vi "SMS Image Preview.vi"(7 "Calling VI Ref":refnum<vi>) -> ()   [LabVIEW 2016]
uses:
  <vilib>/Utility/miscctls.llb/LVPointTypeDef.ctl
  Hardware Configuration/Hardware Configuration Controls/Device Function.ctl
  SMS Image Preview Type Defs/SMS Image Preview Notifier Type.ctl
  SMS Image Preview Type Defs/SMS Image Preview Actions.ctl
  <vilib>/vision/Image Controls.llb/IMAQ Image.ctl
  Device Library/Cameras/Hamamatsu/Orca Flash/Orca Flash Controls/Orca Flash Actions.ctl
  Hardware Configuration/Hardware Configuration Controls/Device Type.ctl
  Device Library/FPGA/FPGA Controls/FPGA Action.ctl
  Device Library/Cameras/Camera Controls/Camera IMAQ Key Info.ctl
  Device Library/Lasers/Laser Controls/Laser Actions.ctl
  Device Library/Lasers/Laser Controls/Laser Settings.ctl
  Device Library/Lasers/Laser Controls/Laser Parameters.ctl
  <vilib>/Analysis/baseanly.llb/Mean (DBL).vi
  <vilib>/vision/NI_Vision_Development_Module.lvlib
  <vilib>/Analysis/NI_AALBase.lvlib
panel:
  in  "YOffset":i32
  in  "XOffset":i32
  in  "Angle (degrees)":sgl format="%.2f"
  out "Current Emitter No.":u16
  in  "Duration":u32 max=65535 step=1
  in  "P Const.":dbl=0.5
  in  "Target Emitter No.":u16=3
  in  "Lock Density":bool
  in  "Average Frame No.":i32=100
  in  "Edge Size":i32=12
  in  "Use Quadrant":bool
  in  "Reset Plot":bool
  out "Blink No. vs. Time":cluster{dbl[], u16[]}(graph)
  in  "Accumulate":bool
  in  "Blink Sensitivity":sgl=10.0
  in  "Image Display":bool
  in  "SMS Preview":bool
  in  "Camera ROI":bool
  in  "Camera":i32(ring) items=["Hamamatsu-Camera-Primary-0"]
  in  "Quit":bool
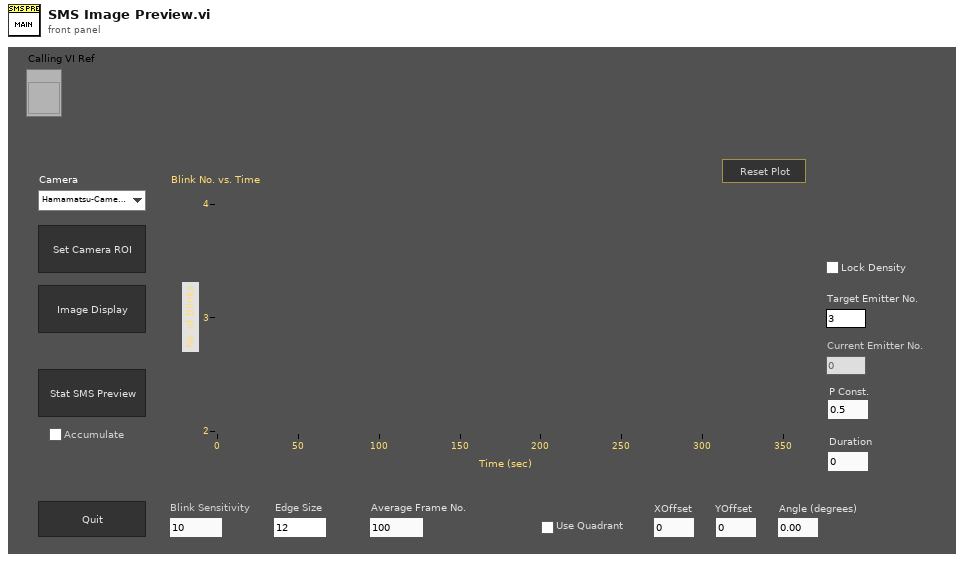
[diagram p1: front panel]
types:
  T1 = typedef "Image Type" = u32
  T2 = typedef "FPGA Action.ctl" = enum16{"Set Laser Mode", "Set Sequence", "Set Duration", "Write Check", "Idle", "Quit"}
  T3 = typedef "Device Function.ctl" = enum16{"Primary", "Secondary", "Overview", "Wide Field Drift Correction", "642 nm Excitation", "560 nm Excitation", "940 nm Excitation", "546 nm Excitation", "488 nm Excitation", "405 nm Excitation", "Objective Drift Correction", "4Pi Focus Lock", "4Pi Objective Lock", "Objective XY", "Objective Z", "Sample XY", "Sample Coarse Z", "Sample Z", "4Pi Lower", "4Pi Upper", "Em Small", "Em Large", "Ex Small", "Ex Large", "Mojo", "Adj Cavity", "Line Scanning", "Alert"}
  T4 = typedef "Device Type.ctl" = enum16{"AOTF", "Camera", "Deformable Mirror", "Laser", "Flip Mirror", "Shutter", "Stage", "Waveform", "FPGA", "Email"}
  T5 = enum8{"Enabled", "Disabled", "Disabled and Grayed Out"}
  T6 = typedef "Orca Flash Actions.ctl" = enum16{"IDLE", "PREVIEW", "RECORD", "Send Trigger", "SOFT TRIGGER", "Record Settings", "SETPARAM", "GETPARAM", "SETROI", "GETROI", "PROGRESSIVE MODE", "AREA MODE", "STATUS", "QUIT"}
  T7 = typedef "SMS Image Preview Actions.ctl" = enum16{"Idle", "Start SMS Preview", "Get Image", "Get Quad", "Sum Quad", "Convolve and Threshold", "Subtract > Dilate", "And Image", "Remove Edge", "Update Plot", "Update Duration", "Abort", "Exit Loop", "Quit"}
  T8 = typedef "SMS Image Preview Notifier Type.ctl" = cluster{"Action":T7, "Camera Notifier Name":string, "Camera Image (U16)":T9, "Camera ROI":cluster{"Global Rectangle":i32[], "Contours":cluster{"Contour Type":u32, "ROI Type":u32, "Points":i32[]}[]}, "SMS Preview (U16)":T9, "Camera ROI (U16)":T9, "Threshold (U16)":T9, "Subtracted > Dilated (U16)":T9, "And Image (U16)":T9, "Camera ROI (SGL)":T9, "Conv 5 x 5 (SGL)":T9, "Conv 11 x 11 (SGL)":T9, "Subtracted (SGL)":T9, "Dilated (SGL)":T9, "Subtracted > Dilated (SGL)":T9, "Ones 5 x 5":sgl[][], "Ones 11 x 11":sgl[][], "Ones 7 x 7":i32[][], "Quads":T9[], "Edge Removed (U16)":T9, "Laser Notifier Name":string, "FPGA Notifier Name":string, "Duration":u32, "Quad 3 TM":T9}
  T9 = typedef "IMAQ Image.ctl" = refnum<image>
  T10 = enum16{"Always On", "Always Off", "Off While Running"}
  T11 = typedef "LVPointTypeDef.ctl" = cluster{"Horizontal":i16, "Vertical":i16}
  T12 = typedef "Camera IMAQ Key Info.ctl" = cluster{"Frame":u32, "Sensor Height":i32, "Sensor Width":i32, "ROI Height":i32, "ROI Width":i32, "ROI Enable?":bool, "Bit per Pixel":u8}
  T13 = enum32{"Average", "Min", "Max", "Clear  if < ", "Clear  if < or =", "Clear  if =", "Clear  if > or =", "Clear  if >"}
  T14 = enum32{"AutoM", "Close", "Dilate", "Erode", "Gradient", "Gradient in", "Gradient out", "HitMiss", "Open", "PClose", "POpen", "Thick", "Thin"}
  T15 = enum32{"Invalid", "Standard", "Closed", "Hidden", "Minimized", "Maximized"}
  T16 = cluster{"Global Rectangle":i32[], "Contours":cluster{"Contour Type":u32, "ROI Type":u32, "Points":i32[]}[]}
  T17 = typedef "Laser Parameters.ctl" = enum16{"Wavelength (nm)", "Pulsing?", "Rep. Rate", "External Control", "Enable Fine", "Fine A", "Fine B", "Channel No."}
  T18 = typedef "Laser Settings.ctl" = cluster{"Laser Parameters":T17, "Value":dbl}
  T19 = typedef "Laser Actions.ctl" = enum16{"Error Check", "Set On/Off", "Set Power", "Set Parameter", "Get Power", "Get Status", "Get Parameter", "Quit"}
  T20 = cluster{"histogram":u32[], "Minimal Value":sgl, "Maximal Value":sgl, "Starting Value":sgl, "Interval Width":sgl, "Mean Value":sgl, "Standard  Variation":sgl, "Area (pixels)":i32}
  T21 = typedef "LVRectTypeDef.ctl" = cluster{"Left":i16, "Top":i16, "Right":i16, "Bottom":i16}
  T22 = typedef "LVBoundsTypeDef.ctl" = cluster{"Width":u32, "Height":u32}
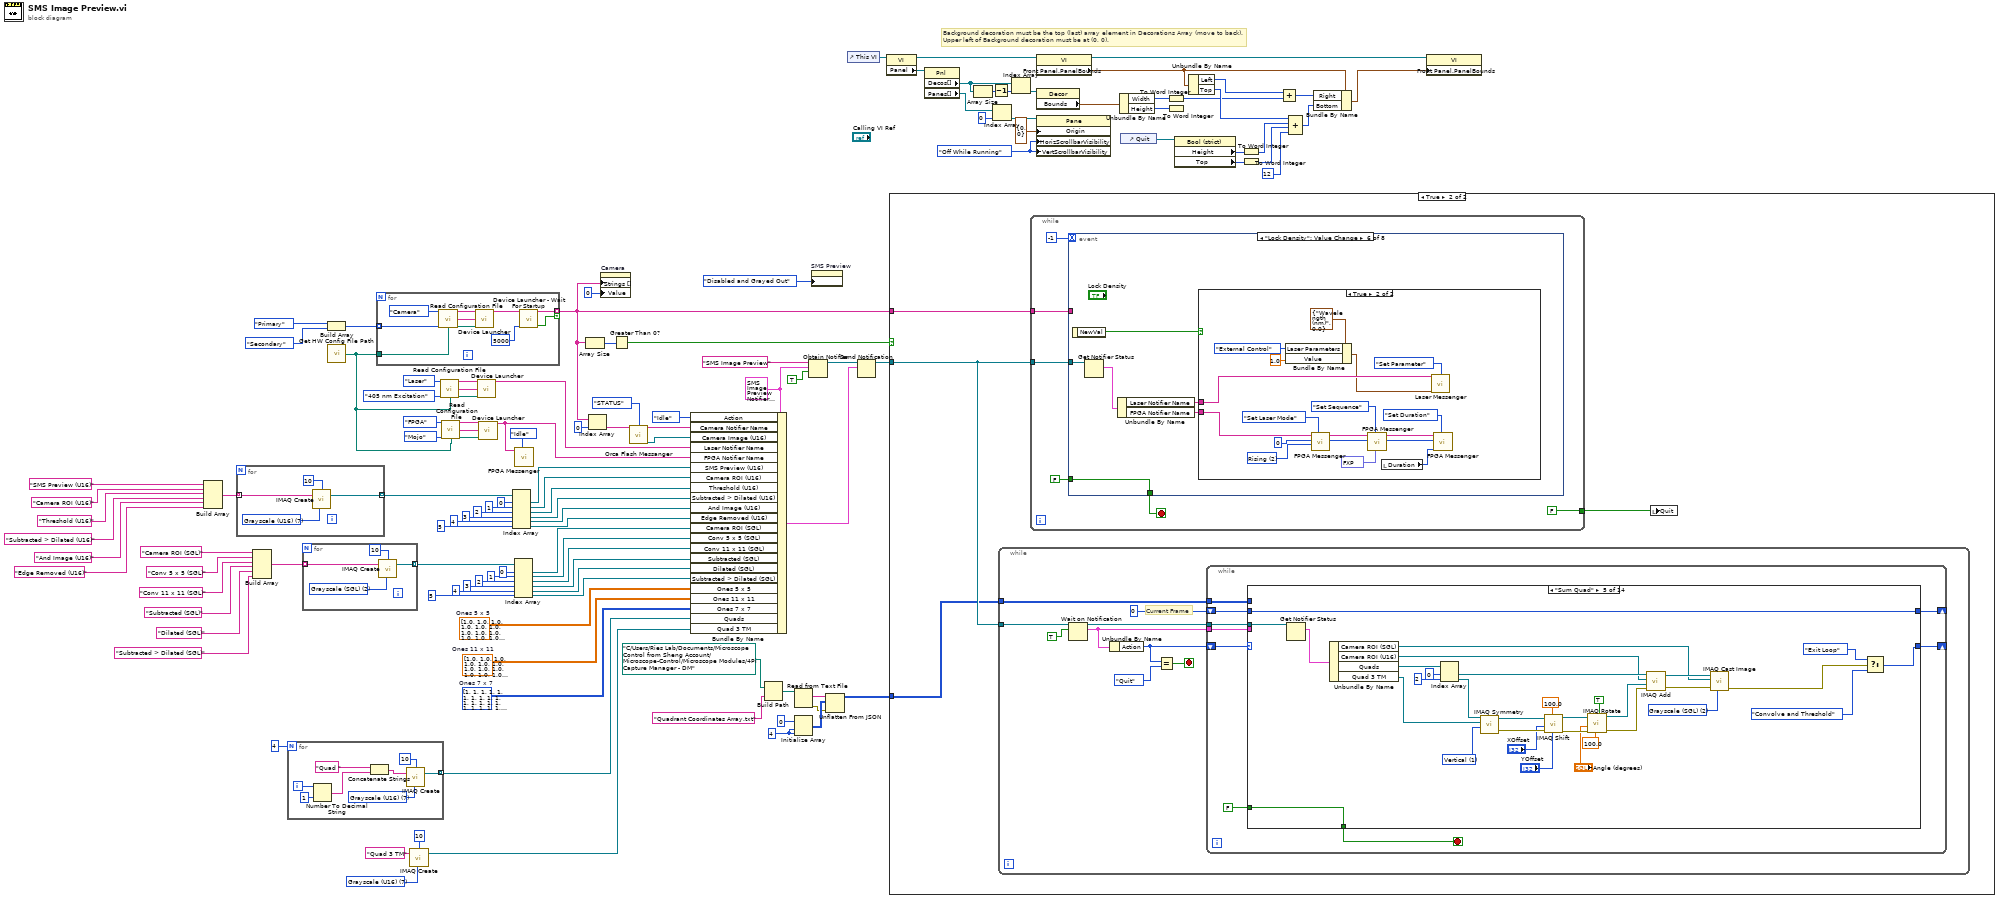
[diagram p0: block diagram]
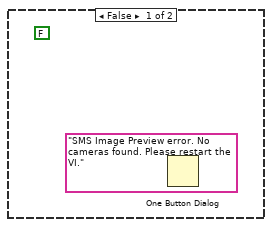
[diagram p2: hidden frame]
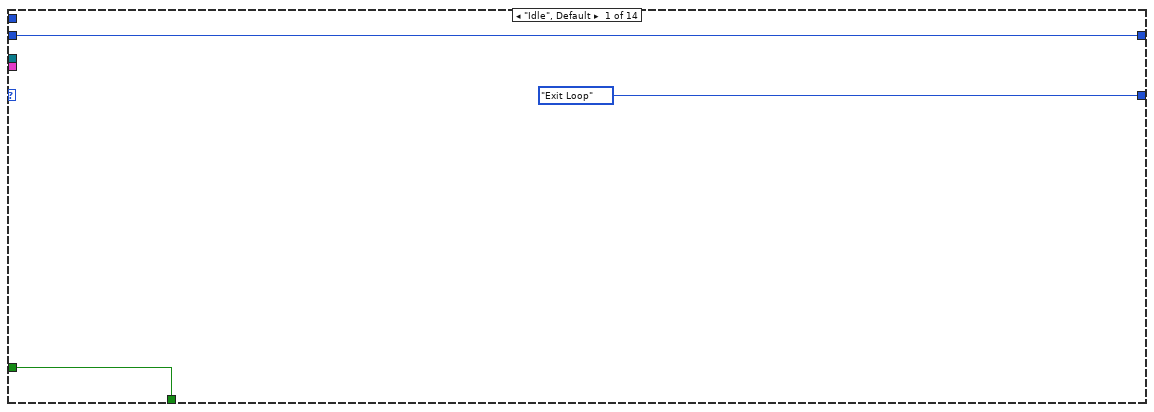
[diagram p3: hidden frame]
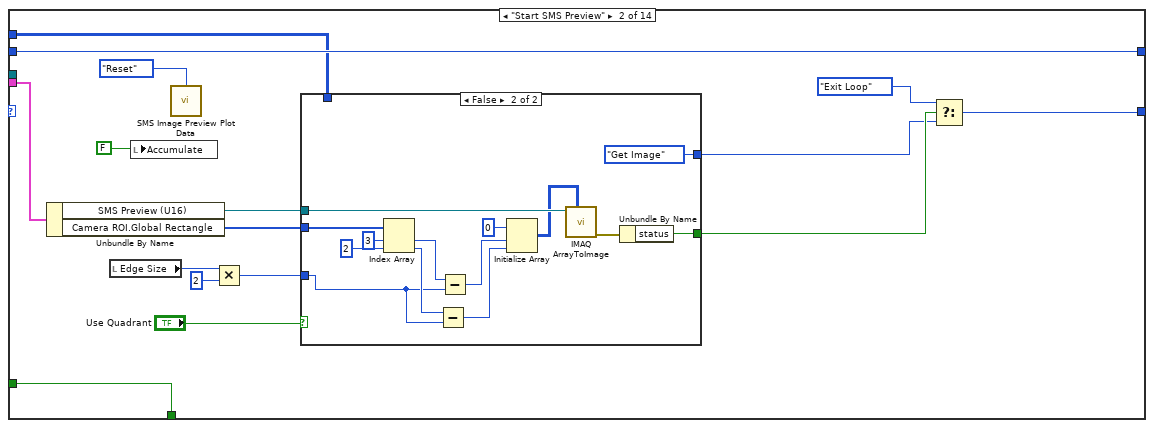
[diagram p4: hidden frame]
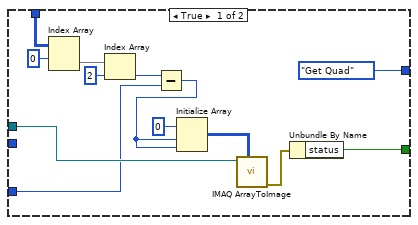
[diagram p5: hidden frame]
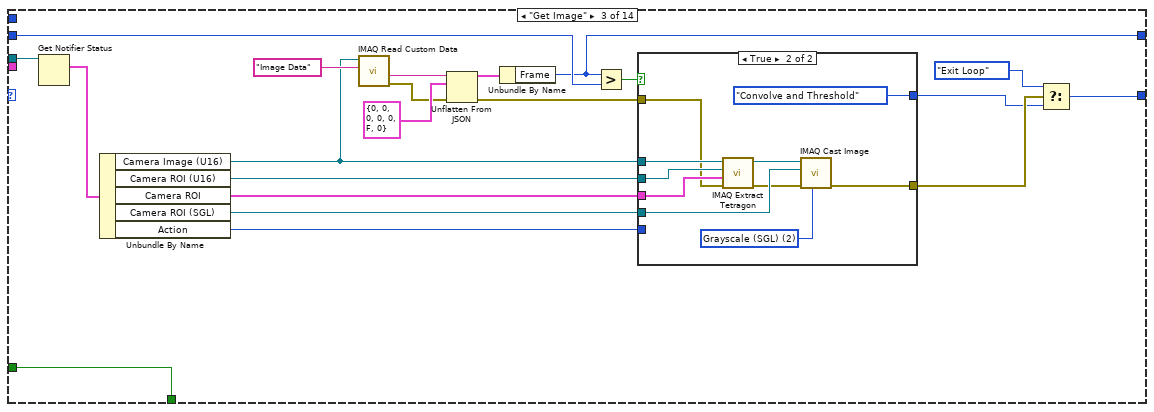
[diagram p6: hidden frame]
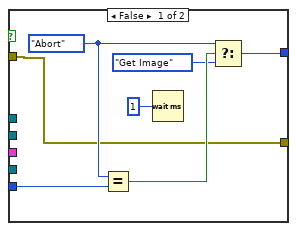
[diagram p7: hidden frame]
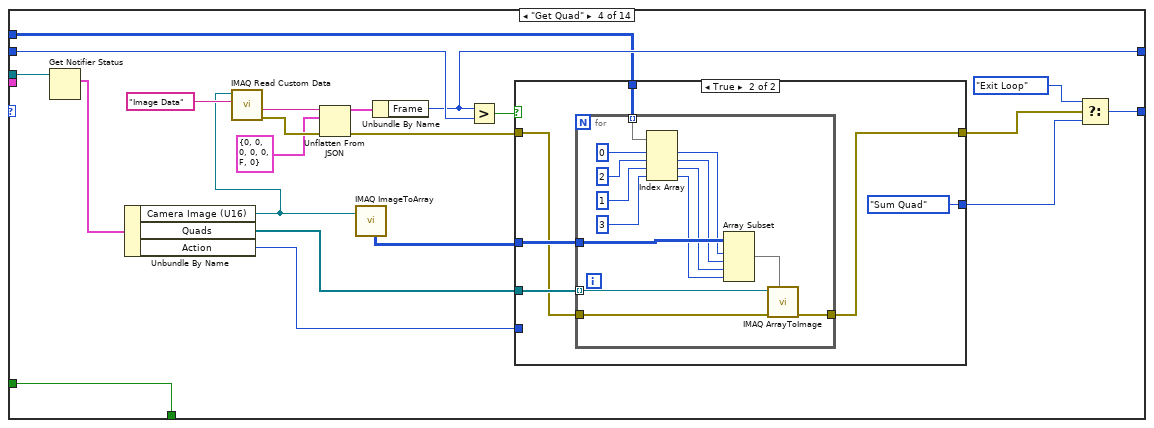
[diagram p8: hidden frame]
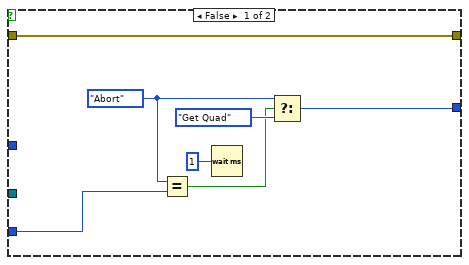
[diagram p9: hidden frame]
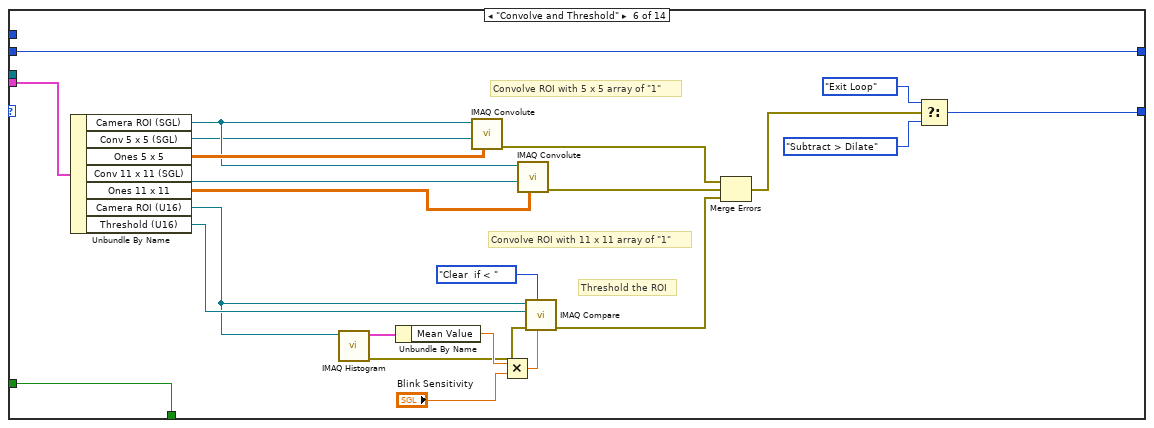
[diagram p10: hidden frame]
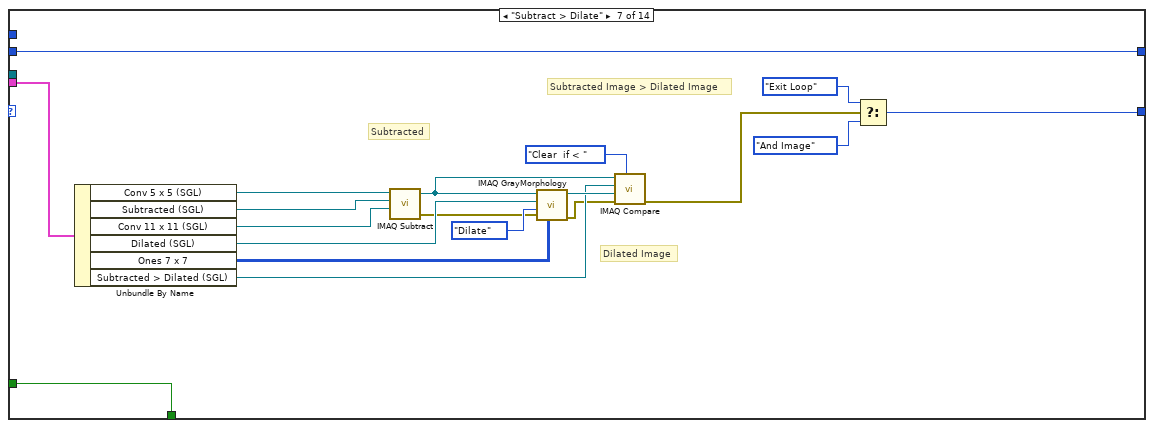
[diagram p11: hidden frame]
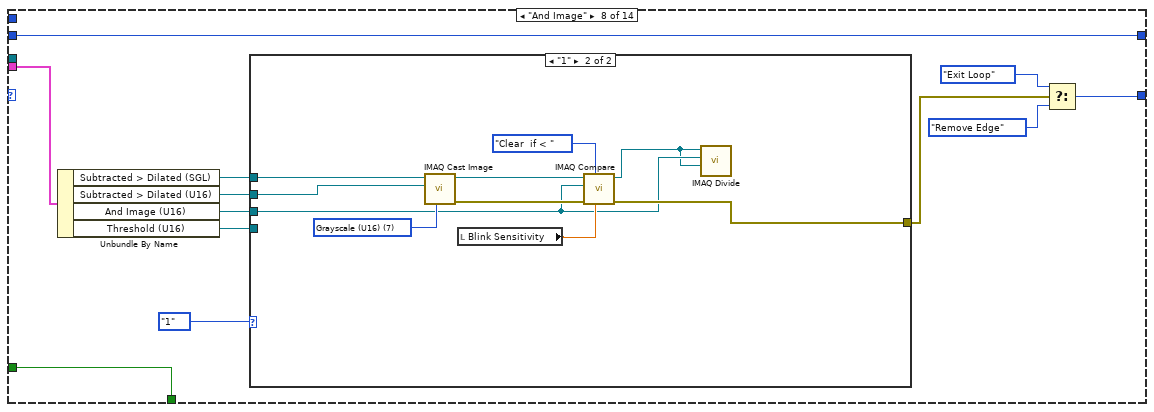
[diagram p12: hidden frame]
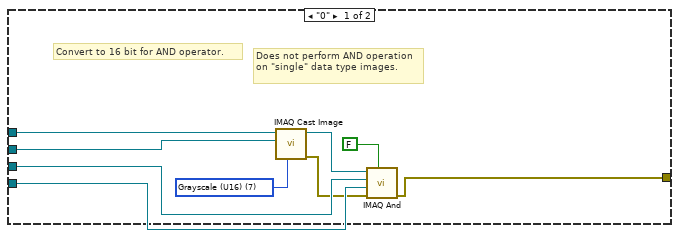
[diagram p13: hidden frame]
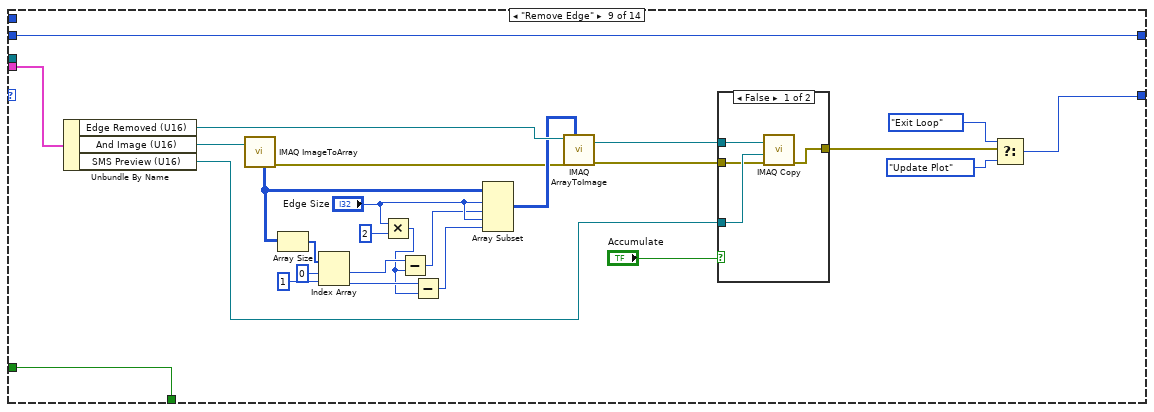
[diagram p14: hidden frame]
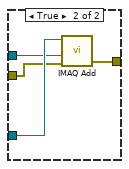
[diagram p15: hidden frame]
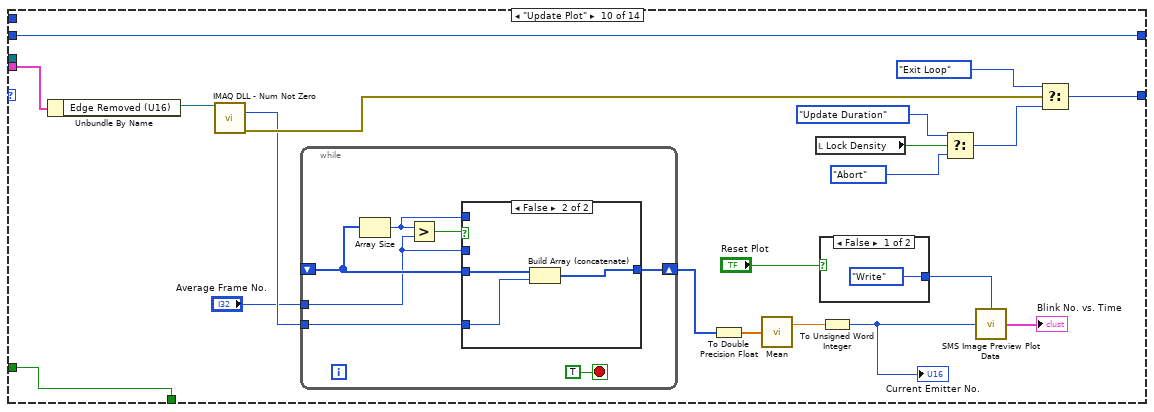
[diagram p16: hidden frame]
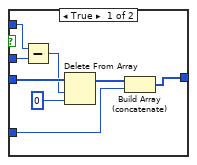
[diagram p17: hidden frame]
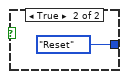
[diagram p18: hidden frame]
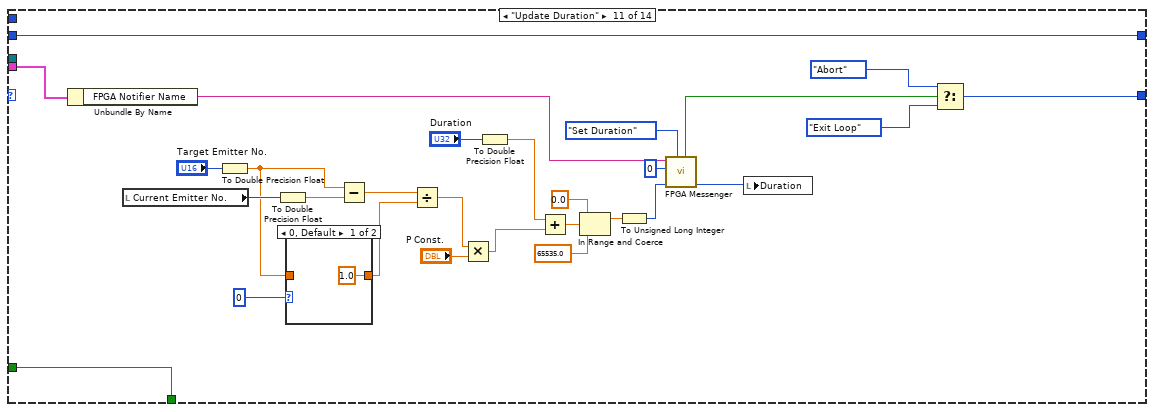
[diagram p19: hidden frame]
diagram:
  w5 = T1 7 items=["Grayscale (U8)", "Grayscale (I16)", "Grayscale (SGL)", "Complex (CSG)", "RGB (U32)", "HSL (U32)", "RGB (U64)", "Grayscale (U16)"] ("Image Type")
  w26 = 4 ("dimension size")
  w37 = i32[][] [[1, 1, 1, 1, 1, 1, 1], [1, 1, 1, 1, 1, 1, 1], [1, 1, 1, 1, 1, 1, 1], [1, 1, 1, 1, 1, 1, 1], [1, 1, 1, 1, 1, 1, 1], [1, 1, 1, 1, 1, 1, 1], [1, 1, 1, 1, 1, 1, 1]]  # Ones 7 x 7
  w38 = sgl[][] [[1.0, 1.0, 1.0, 1.0, 1.0, 1.0, 1.0, 1.0, 1.0, 1.0, 1.0], [1.0, 1.0, 1.0, 1.0, 1.0, 1.0, 1.0, 1.0, 1.0, 1.0, 1.0], [1.0, 1.0, 1.0, 1.0, 1.0, 1.0, 1.0, 1.0, 1.0, 1.0, 1.0], [1.0, 1.0, 1.0, 1.0, 1.0, 1.0, 1.0, 1.0, 1.0, 1.0, 1.0], [1.0, 1.0, 1.0, 1.0, 1.0, 1.0, 1.0, 1.0, 1.0, 1.0, 1.0], [1.0, 1.0, 1.0, 1.0, 1.0, 1.0, 1.0, 1.0, 1.0, 1.0, 1.0], [1.0, 1.0, 1.0, 1.0, 1.0, 1.0, 1.0, 1.0, 1.0, 1.0, 1.0], [1.0, 1.0, 1.0, 1.0, 1.0, 1.0, 1.0, 1.0, 1.0, 1.0, 1.0], [1.0, 1.0, 1.0, 1.0, 1.0, 1.0, 1.0, 1.0, 1.0, 1.0, 1.0], [1.0, 1.0, 1.0, 1.0, 1.0, 1.0, 1.0, 1.0, 1.0, 1.0, 1.0], [1.0, 1.0, 1.0, 1.0, 1.0, 1.0, 1.0, 1.0, 1.0, 1.0, 1.0]]  # Ones 11 x 11
  w39 = sgl[][] [[1.0, 1.0, 1.0, 1.0, 1.0], [1.0, 1.0, 1.0, 1.0, 1.0], [1.0, 1.0, 1.0, 1.0, 1.0], [1.0, 1.0, 1.0, 1.0, 1.0], [1.0, 1.0, 1.0, 1.0, 1.0]]  # Ones 5 x 5
  w34 = T8 {"Action"=enum."Idle", "Camera Notifier Name"="", "Camera Image (U16)"=refnum, "Camera ROI"={"Global Rectangle"=[], "Contours"=[]}, "SMS Preview (U16)"=refnum, "Camera ROI (U16)"=refnum, "Threshold (U16)"=refnum, "Subtracted > Dilated (U16)"=refnum, "And Image (U16)"=refnum, "Camera ROI (SGL)"=refnum, "Conv 5 x 5 (SGL)"=refnum, "Conv 11 x 11 (SGL)"=refnum, "Subtracted (SGL)"=refnum, "Dilated (SGL)"=refnum, "Subtracted > Dilated (SGL)"=refnum, "Ones 5 x 5"=[], "Ones 11 x 11"=[], "Ones 7 x 7"=[], "Quads"=[], "Edge Removed (U16)"=refnum, "Laser Notifier Name"="", "FPGA Notifier Name"="", "Duration"=0, "Quad 3 TM"=refnum} ("SMS Image Preview Notifier Type")
  w104 = T10."Off While Running" ("Vertical Scrollbar Visibility")
  # "Background decoration must be the top (last) array element in Decorations Array (move to back).\nUpper left of Background decoration must be at (0, 0)."
  n1 = Build Array("SMS Preview (U16)" ("Image Name"), "Camera ROI (U16)" ("Image Name"), "Threshold (U16)" ("Image Name"), "Subtracted > Dilated (U16)" ("Image Name"), "And Image (U16)" ("Image Name"), "Edge Removed (U16)" ("element")) -> (w49:string[])
  n2 = for {
    tunnel: w49 -> [w123] mode=indexing
    tunnel: [w122] -> w50 mode=indexing
    w124 = T1 7 items=["Grayscale (U8)", "Grayscale (I16)", "Grayscale (SGL)", "Complex (CSG)", "RGB (U32)", "HSL (U32)", "RGB (U64)", "Grayscale (U16)"] ("Image Type")
    n3 = call "IMAQ Create"("Border Size"=10, "Image Name"=w123, "Image Type"=w124) -> ("New Image"=w122:T9)  [unwired: 2 in, 1 out]
  }
  n4 = Build Array("Camera ROI (SGL)" ("Image Name"), "Conv 5 x 5 (SGL)" ("Image Name"), "Conv 11 x 11 (SGL)" ("Image Name"), "Subtracted (SGL)" ("Image Name"), "Dilated (SGL)" ("Image Name"), "Subtracted > Dilated (SGL)" ("Image Name")) -> (w69:string[])
  n5 = for {
    N: 4 -> [_]
    tunnel: [w131] -> w33 mode=indexing
    i -> [w130]
    w133 = T1 7 items=["Grayscale (U8)", "Grayscale (I16)", "Grayscale (SGL)", "Complex (CSG)", "RGB (U32)", "HSL (U32)", "RGB (U64)", "Grayscale (U16)"] ("Image Type")
    n6 = Number To Decimal String(number=w130, width (-)=i16 1) -> (decimal integer string=w127:string)
    n7 = Concatenate Strings("Quad " ("Image Name"), w127) -> (w126:string)
    n8 = call "IMAQ Create"("Border Size"=10, "Image Name"=w126, "Image Type"=w133) -> ("New Image"=w131:T9)  [unwired: 2 in, 1 out]
  }
  n9 = for {
    tunnel: w69 -> [w135] mode=indexing
    tunnel: [w134] -> w68 mode=indexing
    w136 = T1 2 items=["Grayscale (U8)", "Grayscale (I16)", "Grayscale (SGL)", "Complex (CSG)", "RGB (U32)", "HSL (U32)", "RGB (U64)", "Grayscale (U16)"] ("Image Type")
    n10 = call "IMAQ Create"("Border Size"=10, "Image Name"=w135, "Image Type"=w136) -> ("New Image"=w134:T9)  [unwired: 2 in, 1 out]
  }
  n11 = Build Array(Device_Function."Primary" ("Device Function"), Device_Function."Secondary" ("Device Function")) -> (w90:T3[])
  n12 = call "Get HW Config File Path.vi"() -> ("File Path"=w8:path)  [unwired: 14 in, 1 out]
  n13 = for {
    tunnel: w90 -> [w143] mode=indexing
    tunnel: w8 -> [w142]
    tunnel: [w140] -> w80 mode=indexing if=w139
    n14 = call "Read Configuration File.vi"("Device Type"=Device_Type."Camera", "Device Function"=w143, "Config File Path"=w142) -> ("Unique Notifier Name"=w145:string, "Device Ports/IDs/Channels"=w147:string[], "Device Engine Path"=w146:path)  [unwired: 9 in, 1 out]
    n15 = call "Device Launcher.vi"("Notifier Name"=w145, "Device Ports/IDs/Channels"=w147, "Device Engine Path"=w146) -> ("Notifier Name"=w141:string)  [unwired: 11 in, 1 out]
    n16 = call "Device Launcher - Wait For Startup.vi"("Notifier Name"=w141, "Wait Time (ms)"=5000) -> ("Notifier Name (Dup)"=w140:string, "Running?"=w139:bool)  [unwired: 12 in]
  }
  n17 = call "IMAQ Create"("Border Size"=10, "Image Name"="Quad 3 TM", "Image Type"=w5) -> ("New Image"=w2:T9)  [unwired: 2 in, 1 out]
  n18 = call "Read Configuration File.vi"("Device Type"=Device_Type."Laser", "Device Function"=Device_Function."405 nm Excitation", "Config File Path"=w8) -> ("Unique Notifier Name"=w17:string, "Device Ports/IDs/Channels"=w16:string[], "Device Engine Path"=w15:path)  [unwired: 9 in, 1 out]
  n19 = call "Read Configuration File.vi"("Device Type"=Device_Type."FPGA", "Device Function"=Device_Function."Mojo", "Config File Path"=w8) -> ("Unique Notifier Name"=w11:string, "Device Ports/IDs/Channels"=w10:string[], "Device Engine Path"=w9:path)  [unwired: 9 in, 1 out]
  n20 = call "Device Launcher.vi"("Notifier Name"=w17, "Device Ports/IDs/Channels"=w16, "Device Engine Path"=w15) -> ("Notifier Name"=w14:string)  [unwired: 11 in, 1 out]
  n21 = call "Device Launcher.vi"("Notifier Name"=w11, "Device Ports/IDs/Channels"=w10, "Device Engine Path"=w9) -> ("Notifier Name"=w7:string)  [unwired: 11 in, 1 out]
  n22 = Index Array(array=w50, index #1=0 ("index"), index #2=1 ("index"), index #3=2 ("index"), index #4=3 ("index"), index #5=4 ("index"), index #6=5 ("index")) -> (element #1=w48:T9, element #2=w47:T9, element #3=w46:T9, element #4=w22:T9, element #5=w21:T9, element #6=w20:T9)
  n23 = Index Array(array=w68, index #1=0 ("index"), index #2=1 ("index"), index #3=2 ("index"), index #4=3 ("index"), index #5=4 ("index"), index #6=5 ("index")) -> (element #1=w45:T9, element #2=w44:T9, element #3=w43:T9, element #4=w42:T9, element #5=w41:T9, element #6=w40:T9)
  n24 = call "FPGA Messenger.vi"("FPGA Action"=FPGA_Action."Idle", "Notifier Name"=w7) -> ()  [unwired: 4 in, 6 out]
  n25 = Array Size(array=w80) -> (size(s)=w89:i32)
  n26 = Index Array(array=w80, index=0) -> (element=w78:string)
  n27 = property on="Camera" class="Ring (strict)"("Strings []"=w80, "Value"=0) -> ()  [unwired: 2 in, 2 out]
  n28 = Greater Than 0?(x=w89) -> (x > 0?=w88:bool)
  n29 = call "Orca Flash Messanger.vi"("Notifier Name"=w78, "Camera Actions"=Orca_Flash_Actions."STATUS") -> ("Notifier Name Dup"=w77:string, "Image Ref"=w75:T9)  [unwired: 9 in, 3 out]
  n30 = Bundle By Name(cluster=w34, "Action"=SMS_Image_Preview_Actions."Idle", "Camera Notifier Name"=w77, "Camera Image (U16)"=w75, "Laser Notifier Name"=w14, "FPGA Notifier Name"=w7, "SMS Preview (U16)"=w48, "Camera ROI (U16)"=w47, "Threshold (U16)"=w46, "Subtracted > Dilated (U16)"=w22, "And Image (U16)"=w21, "Edge Removed (U16)"=w20, "Camera ROI (SGL)"=w45, "Conv 5 x 5 (SGL)"=w44, "Conv 11 x 11 (SGL)"=w43, "Subtracted (SGL)"=w42, "Dilated (SGL)"=w41, "Subtracted > Dilated (SGL)"=w40, "Ones 5 x 5"=w39, "Ones 11 x 11"=w38, "Ones 7 x 7"=w37, "Quads"=w33, "Quad 3 TM"=w2) -> (w81:T8)
  n31 = Build Path(base path=path "C:/Users/Ries Lab/Documents/Microscope Control from Sheng Account/Microscope-Control/Microscope Modules/4Pi Capture Manager - DM" ("path"), name or relative path="Quadrant Coordinates Array.txt") -> (appended path=w29:path)
  n32 = Read from Text File(file (use dialog)=w29) -> (text=w28:string, error out=w27:errorcluster)  [unwired: 3 in, 2 out]
  n33 = Initialize Array(0 ("element"), w26, w26) -> (w30:i32[][])
  n34 = Obtain Notifier(name (unnamed)="SMS Image Preview", notification data type=w34, create if not found? (T)=TRUE) -> (notifier out=w84:refnum<notifier>)  [unwired: 1 in, 2 out]
  n35 = property on="SMS Preview" class="Bool (strict)"("DisabledEnum"=T5."Disabled and Grayed Out" ("Disabled")) -> ()  [unwired: 2 in, 2 out]
  n36 = Unflatten From JSON(JSON string=w28, type and defaults=w30, error in (no error)=w27) -> (value=w25:i32[][])  [unwired: 4 in, 1 out]
  n37 = control-ref of="This VI"() -> (w96:refnum<vi>)
  n38 = Send Notification(notification=w81, notifier=w84) -> (notifier out=w82:refnum<notifier>)  [unwired: 1 in, 1 out]
  n39 = property class="VI"(reference=w96) -> (reference out=w105:refnum<vi>, "Panel"=w97:refnum<vi>)  [unwired: 1 in, 1 out]
  n40 = case shown="True" w88 {
    tunnel: w80 -> [_ w152]
    tunnel: w82 -> [_ w150]
    tunnel: w25 -> [_ w149]
    frame False {
      (unwired) FALSE
      n41 = One Button Dialog(message="SMS Image Preview error. No cameras found. Please restart the VI.") -> ()  [unwired: 1 in, 1 out]
    }
    frame True {
      n42 = while {
        tunnel: w150 -> [w161]
        tunnel: w149 -> [w153]
        stop <- w158 stop-if-true
        # "Current Frame"
        n43 = Wait on Notification(notifier=w161, ignore previous (F)=TRUE) -> (notifier out=w154:refnum<notifier>, notification=w156:T8)  [unwired: 2 in, 2 out]
        n44 = Unbundle By Name(w156) -> ("Action"=w157:T7)
        n45 = Equal?(x=w157, y=SMS_Image_Preview_Actions."Quit") -> (x = y?=w158:bool)
        n46 = while {
          shift-right: [w162] -> _
          shift-left: w157 -> [w170]
          tunnel: w156 -> [w169]
          shift-right: [w167] -> _
          shift-left: u32 0 -> [w168]
          tunnel: w154 -> [w166]
          tunnel: w153 -> [w163]
          stop <- w164 stop-if-true
          n47 = case shown="\"Sum Quad\"" w170 {
            tunnel: w169 -> [_ w187 _ _ _ w356 w375 w387 w423 w458 w498 _ _ _]
            tunnel: [SMS_Image_Preview_Actions."Exit Loop" ("y") w184 w219 w257 w312 w337 w358 w378 w415 w460 w500 w517 SMS_Image_Preview_Actions."Exit Loop" ("f") SMS_Image_Preview_Actions."Quit" ("f")] -> w162
            tunnel: w168 -> [w172 w189 w233 w266 w323 w357 w376 w388 w418 w461 w504 w522 w528 w545]
            tunnel: [w172 w189 w232 w265 w323 w357 w376 w388 w418 w461 w504 w522 w528 w545] -> w167
            tunnel: w166 -> [_ _ w227 w274 w324 _ _ _ _ _ _ w521 _ w542]
            tunnel: FALSE -> [w171 w188 w228 w275 w311 w347 w364 w382 w414 w453 w499 w515 _ _]
            tunnel: [w171 w188 w228 w275 w311 w347 w364 w382 w414 w453 w499 w515 TRUE TRUE] -> w164
            tunnel: w163 -> [_ w178 _ w256 _ _ _ _ _ _ _ _ _ _]
            frame "Idle", Default {
            }
            frame "Start SMS Preview" {
              n48 = Unbundle By Name(w187) -> ("SMS Preview (U16)"=w185:T9, "Camera ROI.Global Rectangle"=w186:i32[])
              n49 = local read "Edge Size"() -> (w176:i32)
              n50 = local write "Accumulate"(FALSE ("Accumulate")) -> ()
              n51 = call "SMS Image Preview Plot Data.vi"("Plot Data Actions"=enum16{"Read", "Write", "Reset"}."Reset") -> ()  [unwired: 14 in, 1 out]
              n52 = Multiply(x=w176, y=2) -> (x*y=w174:i32)
              n53 = case shown="False" "Use Quadrant" {
                tunnel: w186 -> [_ w216]
                tunnel: w185 -> [w193 w212]
                tunnel: [w199 w209] -> w183
                tunnel: [SMS_Image_Preview_Actions."Get Quad" ("y") SMS_Image_Preview_Actions."Get Image" ("y")] -> w179
                tunnel: w178 -> [w197 _]
                tunnel: w174 -> [w191 w204]
                frame True {
                  n54 = Index Array(array=w197, index (row)=0) -> (element=w195:i32[])  [unwired: 1 in]
                  n55 = Index Array(array=w195, index=2) -> (element=w192:i32)
                  n56 = Subtract(x=w192, y=w191) -> (x-y=w190:i32)
                  n57 = Initialize Array(u16 0 ("index"), w190, w190) -> (w201:u16[][])
                  n58 = call "IMAQ ArrayToImage"("Image Pixels (U16)"=w201, "Image"=w193) -> ("error out"=w202:errorcluster)  [unwired: 8 in, 1 out]
                  n59 = Unbundle By Name(w202) -> ("status"=w199:bool)
                }
                frame False {
                  n60 = Index Array(array=w216, index #1=3 ("index"), index #2=2 ("index")) -> (element #1=w207:i32, element #2=w205:i32)
                  n61 = Subtract(x=w205, y=w204) -> (x-y=w203:i32)
                  n62 = Subtract(x=w207, y=w204) -> (x-y=w206:i32)
                  n63 = Initialize Array(u16 0 ("index"), w206, w203) -> (w211:u16[][])
                  n64 = call "IMAQ ArrayToImage"("Image Pixels (U16)"=w211, "Image"=w212) -> ("error out"=w210:errorcluster)  [unwired: 8 in, 1 out]
                  n65 = Unbundle By Name(w210) -> ("status"=w209:bool)
                }
              }
              n66 = Select(t=SMS_Image_Preview_Actions."Exit Loop", s=w183, f=w179) -> (s? t:f=w184:T7)
            }
            frame "Get Image" {
              n67 = Get Notifier Status(notifier=w227) -> (current notification=w226:T8)  [unwired: 1 in, 4 out]
              n68 = Unbundle By Name(w226) -> ("Camera Image (U16)"=w230:T9, "Camera ROI (U16)"=w229:T9, "Camera ROI"=w217:T16, "Camera ROI (SGL)"=w224:T9, "Action"=w225:T7)
              n69 = call "IMAQ Read Custom Data"("Key"="Image Data", "Image"=w230) -> ("error out"=w223:errorcluster, "Custom Data Out"=w235:string)  [unwired: 7 in, 1 out]
              n70 = Unflatten From JSON(JSON string=w235, type and defaults=T12 {"Frame"=0, "Sensor Height"=0, "Sensor Width"=0, "ROI Height"=0, "ROI Width"=0, "ROI Enable?"=FALSE, "Bit per Pixel"=0} ("Camera IMAQ Key Info"), error in (no error)=w223) -> (value=w237:T12, error out=w222:errorcluster)  [unwired: 4 in]
              n71 = Unbundle By Name(w237) -> ("Frame"=w232:u32)
              n72 = Greater?(x=w232, y=w233) -> (0:w231:bool)
              n73 = case shown="True" w231 {
                tunnel: w230 -> [_ w254]
                tunnel: w229 -> [_ w253]
                tunnel: w217 -> [_ w252]
                tunnel: [w242 SMS_Image_Preview_Actions."Convolve and Threshold" ("y")] -> w220
                tunnel: w225 -> [w244 _]
                tunnel: w224 -> [_ w248]
                tunnel: w222 -> [w238 w247]
                tunnel: [w238 w245] -> w221
                frame False {
                  w243 = SMS_Image_Preview_Actions."Abort" ("x")
                  n74 = Equal?(x=w243, y=w244) -> (x = y?=w241:bool)
                  n75 = Wait (ms)(milliseconds to wait=u32 1) -> ()  [unwired: 1 out]
                  n76 = Select(t=w243, s=w241, f=SMS_Image_Preview_Actions."Get Image" ("y")) -> (s? t:f=w242:T7)
                }
                frame True {
                  w250 = T1 2 items=["Grayscale (U8)", "Grayscale (I16)", "Grayscale (SGL)", "Complex (CSG)", "RGB (U32)", "HSL (U32)", "RGB (U64)", "Grayscale (U16)"] ("Image Type")
                  n77 = call-poly "IMAQ Extract Tetragon"("error in (no error)"=w247, "ROI Descriptor"=w252, "Image Dst"=w253, "Image Src"=w254) -> ("error out"=w246:errorcluster, "Image Dst Out"=w249:T9)  [unwired: 6 in]
                  n78 = call "IMAQ Cast Image"("Image Type"=w250, "error in (no error)"=w246, "Image Dst"=w248, "Image Src"=w249) -> ("error out"=w245:errorcluster)  [unwired: 6 in, 1 out]
                }
              }
              n79 = Select(t=SMS_Image_Preview_Actions."Exit Loop", s=w221, f=w220) -> (s? t:f=w219:T7)
            }
            frame "Get Quad" {
              n80 = Get Notifier Status(notifier=w274) -> (current notification=w273:T8)  [unwired: 1 in, 4 out]
              n81 = Unbundle By Name(w273) -> ("Camera Image (U16)"=w258:T9, "Quads"=w272:T9[], "Action"=w263:T7)
              n82 = call "IMAQ Read Custom Data"("Key"="Image Data", "Image"=w258) -> ("error out"=w271:errorcluster, "Custom Data Out"=w269:string)  [unwired: 7 in, 1 out]
              n83 = Unflatten From JSON(JSON string=w269, type and defaults=T12 {"Frame"=0, "Sensor Height"=0, "Sensor Width"=0, "ROI Height"=0, "ROI Width"=0, "ROI Enable?"=FALSE, "Bit per Pixel"=0} ("Camera IMAQ Key Info"), error in (no error)=w271) -> (value=w267:T12, error out=w261:errorcluster)  [unwired: 4 in]
              n84 = call "IMAQ ImageToArray"("Image"=w258) -> ("Image Pixels (U16)"=w255:u16[][])  [unwired: 3 in, 4 out]
              n85 = Unbundle By Name(w267) -> ("Frame"=w265:u32)
              n86 = Greater?(x=w265, y=w266) -> (0:w264:bool)
              n87 = case shown="True" w264 {
                tunnel: w272 -> [_ w288]
                tunnel: w256 -> [_ w287]
                tunnel: w255 -> [_ w286]
                tunnel: w263 -> [w278 _]
                tunnel: [w277 w284] -> w260
                tunnel: w261 -> [w277 w285]
                tunnel: [w276 SMS_Image_Preview_Actions."Sum Quad" ("y")] -> w259
                frame False {
                  w279 = SMS_Image_Preview_Actions."Abort" ("x")
                  n88 = Equal?(x=w279, y=w278) -> (x = y?=w280:bool)
                  n89 = Wait (ms)(milliseconds to wait=u32 1) -> ()  [unwired: 1 out]
                  n90 = Select(t=w279, s=w280, f=SMS_Image_Preview_Actions."Get Quad" ("y")) -> (s? t:f=w276:T7)
                }
                frame True {
                  n91 = for {
                    tunnel: w288 -> [w301] mode=indexing
                    tunnel: w286 -> [w302]
                    tunnel: w287 -> [w299] mode=indexing
                    tunnel: w285 -> [w290]
                    tunnel: [w289] -> w284
                    n92 = Index Array(array=w299, index #1=0 ("index"), index #2=2 ("index"), index #3=1 ("index"), index #4=3 ("index")) -> (element #1=w297:i32, element #2=w296:i32, element #3=w292:i32, element #4=w291:i32)
                    n93 = Array Subset(array=w302, index (row)=w297, length (row)=w296, index (col)=w292, length (col)=w291) -> (w300:u16[][])
                    n94 = call "IMAQ ArrayToImage"("Image Pixels (U16)"=w300, "error in (no error)"=w290, "Image"=w301) -> ("error out"=w289:errorcluster)  [unwired: 7 in, 1 out]
                  }
                }
              }
              n95 = Select(t=SMS_Image_Preview_Actions."Exit Loop", s=w260, f=w259) -> (s? t:f=w257:T7)
            }
            frame "Sum Quad" {
              w309 = u32 1 items=["Horizontal", "Vertical", "Central", "1st Diagonal", "2nd Diagonal"] ("Type of Symmetry")
              w317 = T1 2 items=["Grayscale (U8)", "Grayscale (I16)", "Grayscale (SGL)", "Complex (CSG)", "RGB (U32)", "HSL (U32)", "RGB (U64)", "Grayscale (U16)"] ("Image Type")
              n96 = Get Notifier Status(notifier=w324) -> (current notification=w322:T8)  [unwired: 1 in, 4 out]
              n97 = Unbundle By Name(w322) -> ("Camera ROI (SGL)"=w316:T9, "Camera ROI (U16)"=w320:T9, "Quads"=w321:T9[], "Quad 3 TM"=w303:T9)
              n98 = Index Array(array=w321, index #1=0 ("index"), index #2=2 ("index")) -> (element #1=w327:T9, element #2=w310:T9)
              n99 = call "IMAQ Symmetry"("Type of Symmetry"=w309, "Image Dst"=w303, "Image Src"=w310) -> ("error out"=w308:errorcluster, "Image Dst Out"=w307:T9)  [unwired: 2 in]
              n100 = call "IMAQ Shift"("YOffset"="YOffset", "Replace Value"=sgl 100.0, "error in (no error)"=w308, "XOffset"="XOffset", "Image Src"=w307) -> ("error out"=w326:errorcluster, "Image Dst Out"=w331:T9)  [unwired: 5 in]
              n101 = call "IMAQ Rotate"("Maintain Size"=TRUE, "Replace Value"=sgl 100.0, "error in (no error)"=w326, "Angle (degrees)"="Angle (degrees)", "Image Src"=w331) -> ("error out"=w325:errorcluster, "Image Dst Out"=w328:T9)  [unwired: 5 in]
              n102 = call "IMAQ Add"("Image Src A"=w327, "Image Dst"=w320, "Image Src B"=w328, "error in (no error)"=w325) -> ("Image Dst Out"=w319:T9, "error out"=w318:errorcluster)  [unwired: 3 in]
              n103 = call "IMAQ Cast Image"("Image Type"=w317, "error in (no error)"=w318, "Image Dst"=w316, "Image Src"=w319) -> ("error out"=w313:errorcluster)  [unwired: 6 in, 1 out]
              n104 = Select(t=SMS_Image_Preview_Actions."Exit Loop", s=w313, f=SMS_Image_Preview_Actions."Convolve and Threshold") -> (s? t:f=w312:T7)
            }
            frame "Convolve and Threshold" {
              # "Threshold the ROI"
              # "Convolve ROI with 11 x 11 array of \"1\""
              # "Convolve ROI with 5 x 5 array of \"1\""
              n105 = Unbundle By Name(w356) -> ("Camera ROI (SGL)"=w349:T9, "Conv 5 x 5 (SGL)"=w346:T9, "Ones 5 x 5"=w355:sgl[][], "Conv 11 x 11 (SGL)"=w345:T9, "Ones 11 x 11"=w354:sgl[][], "Camera ROI (U16)"=w344:T9, "Threshold (U16)"=w348:T9)
              n106 = call "IMAQ Histogram"("Image"=w344) -> ("error out"=w335:errorcluster, "Histogram Report"=w351:T20)  [unwired: 9 in]
              n107 = Unbundle By Name(w351) -> ("Mean Value"=w352:sgl)
              n108 = call "IMAQ Convolute"("Kernel"=w355, "Image Dst"=w346, "Image Src"=w349) -> ("error out"=w342:errorcluster)  [unwired: 7 in, 1 out]
              n109 = Multiply(x=w352, y="Blink Sensitivity") -> (x*y=w353:sgl)
              n110 = call "IMAQ Convolute"("Kernel"=w354, "Image Dst"=w345, "Image Src"=w349) -> ("error out"=w341:errorcluster)  [unwired: 7 in, 1 out]
              n111 = call "IMAQ Compare"("Constant"=w353, "Operator"=T13."Clear  if < ", "error in (no error)"=w335, "Image Dst"=w348, "Image Src A"=w344) -> ("error out"=w340:errorcluster)  [unwired: 5 in, 1 out]
              n112 = Merge Errors(w342, w341, w340) -> (w339:errorcluster)
              n113 = Select(t=SMS_Image_Preview_Actions."Exit Loop", s=w339, f=SMS_Image_Preview_Actions."Subtract > Dilate" ("y")) -> (s? t:f=w337:T7)
            }
            frame "Subtract > Dilate" {
              # "Subtracted Image > Dilated Image"
              # "Subtracted"
              # "Dilated Image"
              n114 = Unbundle By Name(w375) -> ("Conv 5 x 5 (SGL)"=w374:T9, "Subtracted (SGL)"=w373:T9, "Conv 11 x 11 (SGL)"=w372:T9, "Dilated (SGL)"=w369:T9, "Ones 7 x 7"=w370:i32[][], "Subtracted > Dilated (SGL)"=w365:T9)
              n115 = call "IMAQ Subtract"("Image Src A"=w374, "Image Dst"=w373, "Image Src B"=w372) -> ("Image Dst Out"=w366:T9, "error out"=w363:errorcluster)  [unwired: 4 in]
              n116 = call "IMAQ GrayMorphology"("Structuring Element"=w370, "error in (no error)"=w363, "Operation"=T14."Dilate", "Image Dst"=w369, "Image Src"=w366) -> ("error out"=w362:errorcluster, "Image Dst Out"=w367:T9)  [unwired: 5 in]
              n117 = call "IMAQ Compare"("Operator"=T13."Clear  if < ", "error in (no error)"=w362, "Image Src B"=w367, "Image Dst"=w365, "Image Src A"=w366) -> ("error out"=w361:errorcluster)  [unwired: 5 in, 1 out]
              n118 = Select(t=SMS_Image_Preview_Actions."Exit Loop", s=w361, f=SMS_Image_Preview_Actions."And Image" ("y")) -> (s? t:f=w358:T7)
            }
            frame "And Image" {
              n119 = Unbundle By Name(w387) -> ("Subtracted > Dilated (SGL)"=w386:T9, "Subtracted > Dilated (U16)"=w385:T9, "And Image (U16)"=w384:T9, "Threshold (U16)"=w383:T9)
              n120 = case shown="\"1\"" enum16{"0", "1"}."1" {
                tunnel: w386 -> [w395 w405]
                tunnel: w385 -> [w394 w404]
                tunnel: w384 -> [w392 w399]
                tunnel: w383 -> [w391 _]
                tunnel: [w389 w400] -> w379
                frame "0" {
                  w396 = T1 7 items=["Grayscale (U8)", "Grayscale (I16)", "Grayscale (SGL)", "Complex (CSG)", "RGB (U32)", "HSL (U32)", "RGB (U64)", "Grayscale (U16)"] ("Image Type")
                  # "Convert to 16 bit for AND operator."
                  # "Does not perform AND operation on \"single\" data type images."
                  n121 = call "IMAQ Cast Image"("Image Type"=w396, "Image Dst"=w394, "Image Src"=w395) -> ("error out"=w390:errorcluster, "Image Dst Out"=w393:T9)  [unwired: 7 in]
                  n122 = call "IMAQ And"("And/Nand (And)"=FALSE, "error in (no error)"=w390, "Image Src B"=w391, "Image Dst"=w392, "Image Src A"=w393) -> ("error out"=w389:errorcluster)  [unwired: 5 in, 1 out]
                }
                frame "1" {
                  w401 = T1 7 items=["Grayscale (U8)", "Grayscale (I16)", "Grayscale (SGL)", "Complex (CSG)", "RGB (U32)", "HSL (U32)", "RGB (U64)", "Grayscale (U16)"] ("Image Type")
                  n123 = call "IMAQ Cast Image"("Image Type"=w401, "Image Dst"=w404, "Image Src"=w405) -> ("error out"=w402:errorcluster, "Image Dst Out"=w403:T9)  [unwired: 7 in]
                  n124 = local read "Blink Sensitivity"() -> (w406:sgl)
                  n125 = call "IMAQ Compare"("Constant"=w406, "Operator"=T13."Clear  if < ", "error in (no error)"=w402, "Image Dst"=w399, "Image Src A"=w403) -> ("error out"=w400:errorcluster, "Image Dst Out"=w398:T9)  [unwired: 5 in]
                  n126 = call "IMAQ Divide"("Image Src A"=w398, "Image Dst"=w399, "Image Src B"=w398) -> ()  [unwired: 4 in, 2 out]
                }
              }
              n127 = Select(t=SMS_Image_Preview_Actions."Exit Loop", s=w379, f=SMS_Image_Preview_Actions."Remove Edge" ("y")) -> (s? t:f=w378:T7)
            }
            frame "Remove Edge" {
              n128 = Unbundle By Name(w423) -> ("Edge Removed (U16)"=w422:T9, "And Image (U16)"=w432:T9, "SMS Preview (U16)"=w410:T9)
              n129 = call "IMAQ ImageToArray"("Image"=w432) -> ("Image Pixels (U16)"=w424:u16[][], "error out"=w419:errorcluster)  [unwired: 3 in, 3 out]
              n130 = Array Size(array=w424) -> (size(s)=w425:i32[])
              n131 = Index Array(array=w425, index #1=0 ("index"), index #2=1 ("index")) -> (element #1=w429:i32, element #2=w430:i32)
              n132 = Multiply(x="Edge Size", y=2) -> (x*y=w413:i32)
              n133 = Subtract(x=w429, y=w413) -> (x-y=w428:i32)
              n134 = Subtract(x=w430, y=w413) -> (x-y=w427:i32)
              n135 = Array Subset(array=w424, index (row)="Edge Size", length (row)=w428, index (col)="Edge Size", length (col)=w427) -> (w421:u16[][])
              n136 = call "IMAQ ArrayToImage"("Image Pixels (U16)"=w421, "error in (no error)"=w419, "Image"=w422) -> ("error out"=w412:errorcluster, "Image Out"=w411:T9)  [unwired: 7 in]
              n137 = case shown="False" "Accumulate" {
                tunnel: w411 -> [w437 w440]
                tunnel: w410 -> [w436 w441]
                tunnel: w412 -> [w435 w439]
                tunnel: [w434 w438] -> w409
                frame False {
                  n138 = call "IMAQ Copy"("error in (no error)"=w435, "Image Dst"=w436, "Image Src"=w437) -> ("error out"=w434:errorcluster)  [unwired: 3 in, 1 out]
                }
                frame True {
                  n139 = call "IMAQ Add"("Image Src A"=w441, "Image Src B"=w440, "error in (no error)"=w439) -> ("error out"=w438:errorcluster)  [unwired: 4 in, 1 out]
                }
              }
              n140 = Select(t=SMS_Image_Preview_Actions."Exit Loop", s=w409, f=SMS_Image_Preview_Actions."Update Plot" ("y")) -> (s? t:f=w415:T7)
            }
            frame "Update Plot" {
              n141 = Unbundle By Name(w458) -> ("Edge Removed (U16)"=w452:T9)
              n142 = call "IMAQ DLL - Num Not Zero.vi"("IMAQ Ref"=w452) -> ("Non Zero Px Total"=w454:u16, "Error Out"=w457:errorcluster)  [unwired: 12 in, 1 out]
              n143 = while {
                tunnel: w454 -> [w467]
                shift-right: [w466] -> w451
                shift-left: _ -> [w465]
                tunnel: "Average Frame No." -> [w463]
                stop <- TRUE ("stop") stop-if-true
                n144 = Array Size(array=w465) -> (size(s)=w462:i32)
                n145 = Greater?(x=w462, y=w463) -> (0:w464:bool)
                n146 = case shown="False" w464 {
                  tunnel: w467 -> [w473 w479]
                  tunnel: [w472 w478] -> w466
                  tunnel: w465 -> [w476 w477]
                  tunnel: w463 -> [w471 _]
                  tunnel: w462 -> [w470 _]
                  frame True {
                    n147 = Subtract(x=w470, y=w471) -> (x-y=w469:i32)
                    n148 = Delete From Array(array=w476, length=w469, index=0) -> (array with subset deleted=w474:u16[])  [unwired: 1 out]
                    n149 = Build Array (concatenate)(w474, w473) -> (w472:u16[])
                  }
                  frame False {
                    n150 = Build Array (concatenate)(w477, w479) -> (w478:u16[])
                  }
                }
              }
              n151 = To Double Precision Float(number=w451) -> (double precision float=w450:dbl[])
              n152 = call-poly <vilib>:"Mean.vi"("X"=w450) -> ("mean"=w449:dbl)  [unwired: 1 out]
              n153 = local read "Lock Density"() -> (w447:bool)
              n154 = case shown="False" "Reset Plot" {
                tunnel: [enum16{"Read", "Write", "Reset"}."Write" ("Plot Data Actions") enum16{"Read", "Write", "Reset"}."Reset" ("Plot Data Actions")] -> w456
                frame False {
                }
                frame True {
                }
              }
              n155 = To Unsigned Word Integer(number=w449) -> (unsigned 16bit integer=w442:u16)
              "Current Emitter No." <- w442
              n156 = Select(t=SMS_Image_Preview_Actions."Update Duration", s=w447, f=SMS_Image_Preview_Actions."Abort" ("y")) -> (s? t:f=w444:T7)
              n157 = call "SMS Image Preview Plot Data.vi"("Plot Data Actions"=w456, "Blink Number"=w442) -> ("Plot Data"=→"Blink No. vs. Time":cluster{dbl[], u16[]})  [unwired: 13 in]
              n158 = Select(t=SMS_Image_Preview_Actions."Exit Loop" ("y"), s=w457, f=w444) -> (s? t:f=w460:T7)
            }
            frame "Update Duration" {
              n159 = Unbundle By Name(w498) -> ("FPGA Notifier Name"=w507:string)
              n160 = local read "Current Emitter No."() -> (w488:u16)
              n161 = To Double Precision Float(number="Target Emitter No.") -> (double precision float=w482:dbl)
              n162 = To Double Precision Float(number=w488) -> (double precision float=w487:dbl)
              n163 = case shown="0, Default" 0 {
                tunnel: [1.0 w511] -> w485
                tunnel: w482 -> [_ w511]
                frame 0, Default {
                }
                frame 1 {
                }
              }
              n164 = Subtract(x=w482, y=w487) -> (x-y=w486:dbl)
              n165 = Divide(x=w486, y=w485) -> (x/y=w509:dbl)
              n166 = Multiply(x=w509, y="P Const.") -> (x*y=w484:dbl)
              n167 = To Double Precision Float(number="Duration") -> (double precision float=w493:dbl)
              n168 = Add(x=w493, y=w484) -> (x+y=w496:dbl)
              n169 = In Range and Coerce(upper limit=0.0, x=w496, lower limit=65535.0) -> (coerced(x)=w490:dbl)  [unwired: 1 out]
              n170 = To Unsigned Long Integer(number=w490) -> (unsigned 32bit integer=w489:u32)
              n171 = call "FPGA Messenger.vi"("FPGA Action"=FPGA_Action."Set Duration" ("Action"), "Duration"=w489, "Laser Channel"=u16 0, "Notifier Name"=w507) -> ("Duration"=w497:u32, "Write Confirm"=w502:bool)  [unwired: 2 in, 4 out]
              n172 = local write "Duration"(w497) -> ()
              n173 = Select(t=SMS_Image_Preview_Actions."Abort" ("y"), s=w502, f=SMS_Image_Preview_Actions."Exit Loop") -> (s? t:f=w500:T7)
            }
            frame "Abort" {
              n174 = Get Notifier Status(notifier=w521) -> (current notification=w520:T8)  [unwired: 1 in, 4 out]
              n175 = Unbundle By Name(w520) -> ("Action"=w519:T7)
              n176 = Equal?(x=SMS_Image_Preview_Actions."Abort" ("y"), y=w519) -> (x = y?=w516:bool)
              n177 = local read "Use Quadrant"() -> (w513:bool)
              n178 = case shown="True" w513 {
                tunnel: [SMS_Image_Preview_Actions."Get Image" ("f") SMS_Image_Preview_Actions."Get Quad" ("f")] -> w512
                frame False {
                }
                frame True {
                }
              }
              n179 = Select(t=SMS_Image_Preview_Actions."Exit Loop", s=w516, f=w512) -> (s? t:f=w517:T7)
            }
            frame "Exit Loop" {
              n180 = local write "Duration"(u32 0 ("Duration")) -> ()
            }
            frame "Quit" {
              n181 = Release Notifier(notifier=w542) -> (last notification=w541:T8)  [unwired: 2 in, 2 out]
              n182 = Unbundle By Name(w541) -> ("SMS Preview (U16)"=w540:T9, "Camera ROI (U16)"=w538:T9, "Threshold (U16)"=w537:T9, "Subtracted > Dilated (U16)"=w536:T9, "And Image (U16)"=w535:T9, "Camera ROI (SGL)"=w534:T9, "Conv 5 x 5 (SGL)"=w533:T9, "Conv 11 x 11 (SGL)"=w532:T9, "Subtracted (SGL)"=w531:T9, "Dilated (SGL)"=w530:T9, "Subtracted > Dilated (SGL)"=w529:T9)
              n183 = Build Array(w540, w538, w537, w536, w535, w534, w533, w532, w531, w530, w529) -> (w539:T9[])
              n184 = for {
                tunnel: w539 -> [w546] mode=indexing
                n185 = call "IMAQ Dispose"("Image"=w546) -> ()  [unwired: 5 in, 1 out]
              }
            }
          }
        }
      }
      n186 = while {
        tunnel: w152 -> [w549]
        tunnel: w150 -> [w548]
        tunnel: [FALSE] -> w151
        stop <- w550 stop-if-true
        n187 = event shown="[5] \"Lock Density\": Value Change" {
          selector: _ -> [_ _ _ _ _ _ _ _]
          dyn-events: _ -> [_ _ _ _ _ _ _ _]
          timeout: -1 -> [_ _ _ _ _ _ _ _]
          tunnel: FALSE -> [w553 w557 w571 w578 w602 w626 w660 _]
          tunnel: [w553 w557 w571 w578 w602 w626 w660 w666] -> w550
          tunnel: w549 -> [_ _ w570 _ _ _ _ _]
          tunnel: w548 -> [_ _ w568 w577 w586 w629 w659 w665]
          event Timeout {
            n188 = event-data() -> ()  [unwired: 1 in, 1 out]
          }
          event Application Instance Close? {
            n189 = event-data() -> ()  [unwired: 1 in, 1 out]
            n190 = control-ref of="This VI"() -> (w554:refnum<vi>)
            n191 = invoke class="VI" method="FP.Open"(reference=w554, "Activate"=TRUE ("Activate?"), "State"=T15."Standard") -> ()  [unwired: 2 in, 5 out]
            n192 = event-data("Discard?"=TRUE) -> ()  [unwired: 1 in, 1 out]
          }
          event "Camera": Value Change {
            # "Empty ROI"
            n193 = event-data() -> ("NewVal"=w569:i32)  [unwired: 1 in]
            n194 = Index Array(array=w570, index=w569) -> (element=w561:string)
            n195 = call "Orca Flash Messanger.vi"("Notifier Name"=w561, "Camera Actions"=Orca_Flash_Actions."STATUS") -> ("Notifier Name Dup"=w563:string, "Image Ref"=w562:T9)  [unwired: 9 in, 3 out]
            n196 = Get Notifier Status(notifier=w568) -> (notifier out=w567:refnum<notifier>, current notification=w566:T8)  [unwired: 1 in, 3 out]
            n197 = Bundle By Name(cluster=w566, "Action"=SMS_Image_Preview_Actions."Idle", "Camera Notifier Name"=w563, "Camera Image (U16)"=w562, "Camera ROI"=T16 {"Global Rectangle"=[], "Contours"=[]}) -> (w565:T8)
            n198 = Send Notification(notification=w565, notifier=w567) -> ()  [unwired: 1 in, 2 out]
          }
          event "Camera ROI": Value Change {
            n199 = event-data() -> ()  [unwired: 1 in, 1 out]
            n200 = Get Notifier Status(notifier=w577) -> (notifier out=w576:refnum<notifier>, current notification=w572:T8)  [unwired: 1 in, 3 out]
            n201 = Unbundle By Name(w572) -> ("Camera Image (U16)"=w575:T9)
            n202 = call "SMS Image Preview Select ROI.vi"("Camera Image Ref"=w575) -> ("Camera ROI"=w573:T16, "Canceled?"=w574:bool)  [unwired: 13 in]
            n203 = case shown="False" w574 {
              tunnel: w576 -> [w584 _]
              tunnel: w573 -> [w582 _]
              tunnel: w572 -> [w583 _]
              frame False {
                n204 = Bundle By Name(cluster=w583, "Camera ROI"=w582, "Action"=SMS_Image_Preview_Actions."Idle") -> (w581:T8)
                n205 = property on="SMS Preview" class="Bool (strict)"("DisabledEnum"=T5."Enabled" ("Disabled")) -> ()  [unwired: 2 in, 2 out]
                n206 = Send Notification(notification=w581, notifier=w584) -> ()  [unwired: 1 in, 2 out]
              }
              frame True {
              }
            }
          }
          event "Image Display": Value Change {
            n207 = event-data() -> ("NewVal"=w585:bool)  [unwired: 1 in]
            n208 = Get Notifier Status(notifier=w586) -> (current notification=w587:T8)  [unwired: 1 in, 4 out]
            n209 = Unbundle By Name(w587) -> ("SMS Preview (U16)"=w601:T9)
            n210 = Obtain Notifier(name (unnamed)="Display Module IMAQ Refs", notification data type=T9[] [], create if not found? (T)=FALSE) -> (notifier out=w594:refnum<notifier>, error out=w595:errorcluster)  [unwired: 1 in, 1 out]
            n211 = Get Notifier Status(notifier=w594, error in (no error)=w595) -> (notifier out=w593:refnum<notifier>, current notification=w591:T9[], error out=w592:errorcluster)  [unwired: 2 out]
            n212 = case shown="True" w585 {
              tunnel: w593 -> [w610 w623]
              tunnel: w592 -> [w604 w622]
              tunnel: w591 -> [w606 w621]
              tunnel: [w605 w618] -> w588
              tunnel: [w610 w623] -> w590
              tunnel: [w604 w622] -> w589
              tunnel: w601 -> [w603 w620]
              frame False {
                n213 = Equal?(x=w606, y=w603) -> (x = y?=w609:bool[])
                n214 = for {
                  tunnel: w609 -> [w617] mode=indexing
                  tunnel: [w616] -> w607
                  i -> [w616]
                  stop <- w617 stop-if-true
                }
                n215 = Or Array Elements(Boolean array=w609) -> (logical OR=w608:bool)
                n216 = case shown="False" w608 {
                  tunnel: w607 -> [_ w614]
                  tunnel: w606 -> [w611 w613]
                  tunnel: [w611 w612] -> w605
                  frame False {
                  }
                  frame True {
                    n217 = Delete From Array(array=w613, length=1, index=w614) -> (array with subset deleted=w612:T9[])  [unwired: 1 out]
                  }
                }
              }
              frame True {
                n218 = Insert Into Array(array=w621, index=0, new element=w620) -> (w618:T9[])
              }
            }
            n219 = Send Notification(notification=w588, notifier=w590, error in (no error)=w589) -> (notifier out=w596:refnum<notifier>, error out=w597:errorcluster)
            n220 = Release Notifier(notifier=w596, error in (no error)=w597) -> ()  [unwired: 1 in, 3 out]
          }
          event "Lock Density": Value Change {
            n221 = event-data() -> ("NewVal"=w625:bool)  [unwired: 1 in]
            n222 = Get Notifier Status(notifier=w629) -> (current notification=w624:T8)  [unwired: 1 in, 4 out]
            n223 = Unbundle By Name(w624) -> ("Laser Notifier Name"=w628:string, "FPGA Notifier Name"=w627:string)
            n224 = case shown="True" w625 {
              tunnel: w628 -> [_ w651]
              tunnel: w627 -> [w630 w649]
              frame False {
                w631 = u16 0 items=["Off", "On", "Rising", "Falling", "Camera"] ("Laser Mode")
                n225 = call "FPGA Messenger.vi"("FPGA Action"=FPGA_Action."Set Laser Mode" ("Action"), "Laser Mode"=w631, "Laser Channel"=u16 0, "Notifier Name"=w630) -> ()  [unwired: 2 in, 6 out]
              }
              frame True {
                w648 = u16 2 items=["Off", "On", "Rising", "Falling", "Camera"] ("Laser Mode")
                n226 = Bundle By Name(cluster=T18 {"Laser Parameters"=enum."Wavelength (nm)", "Value"=0.0} ("Settings"), "Laser Parameters"=Laser_Parameters."External Control", "Value"=1.0) -> (w634:T18)
                n227 = call "FPGA Messenger.vi"("FPGA Action"=FPGA_Action."Set Laser Mode" ("Action"), "Laser Mode"=w648, "Laser Channel"=u16 0, "Notifier Name"=w649) -> ("Laser Channel"=w643:u16, "Notifier Name Out"=w647:string)  [unwired: 2 in, 4 out]
                n228 = call "FPGA Messenger.vi"("Sequence"=fxp<+,16,16> 65535.0, "FPGA Action"=FPGA_Action."Set Sequence" ("Action"), "Laser Channel"=w643, "Notifier Name"=w647) -> ("Laser Channel"=w642:u16, "Notifier Name Out"=w645:string)  [unwired: 2 in, 4 out]
                n229 = local read "Duration"() -> (w638:u32)
                n230 = call "Laser Messenger.vi"("Notifier Name"=w651, "Action"=Laser_Actions."Set Parameter", "Laser Settings"=w634) -> ()  [unwired: 7 in, 6 out]
                n231 = call "FPGA Messenger.vi"("FPGA Action"=FPGA_Action."Set Duration" ("Action"), "Duration"=w638, "Laser Channel"=w642, "Notifier Name"=w645) -> ()  [unwired: 2 in, 6 out]
              }
            }
          }
          event "SMS Preview": Value Change {
            n232 = event-data() -> ("NewVal"=w655:bool)  [unwired: 1 in]
            n233 = Get Notifier Status(notifier=w659) -> (notifier out=w658:refnum<notifier>, current notification=w657:T8)  [unwired: 1 in, 3 out]
            n234 = Select(t=SMS_Image_Preview_Actions."Start SMS Preview" ("Action"), s=w655, f=SMS_Image_Preview_Actions."Abort") -> (s? t:f=w652:T7)
            n235 = Bundle By Name(cluster=w657, "Action"=w652) -> (w656:T8)
            n236 = Send Notification(notification=w656, notifier=w658) -> ()  [unwired: 1 in, 2 out]
          }
          event "Quit": Value Change {
            n237 = event-data() -> ("NewVal"=w666:bool)  [unwired: 1 in]
            n238 = Get Notifier Status(notifier=w665) -> (notifier out=w663:refnum<notifier>, current notification=w662:T8)  [unwired: 1 in, 3 out]
            n239 = Bundle By Name(cluster=w662, "Action"=SMS_Image_Preview_Actions."Quit") -> (w664:T8)
            n240 = Send Notification(notification=w664, notifier=w663) -> ()  [unwired: 1 in, 2 out]
          }
        }
      }
      n241 = local write "Quit"(w151) -> ()
    }
  }
  n242 = property class="Pnl"(reference=w97) -> ("Decos[]"=w95:refnum<vi>[], "Panes[]"=w101:refnum<vi>[])  [unwired: 1 in, 2 out]
  n243 = Array Size(array=w95) -> (size(s)=w93:i32)
  n244 = Decrement(x=w93) -> (x-1=w94:i32)
  n245 = Index Array(array=w101, index=0) -> (element=w100:refnum<vi>)
  n246 = Index Array(array=w95, index=w94) -> (element=w103:refnum<vi>)
  n247 = property class="VI"(reference=w105) -> (reference out=w107:refnum<vi>, "Front Panel.PanelBounds"=w108:T21)  [unwired: 1 in, 1 out]
  n248 = property class="Decor"(reference=w103) -> ("Bounds"=w106:T22)  [unwired: 1 in, 2 out]
  n249 = property class="Pane"(reference=w100, "Origin"=T11 {"Horizontal"=0, "Vertical"=0}, "HorizScrollbarVisibility"=w104, "VertScrollbarVisibility"=w104) -> ()  [unwired: 1 in, 2 out]
  n250 = Unbundle By Name(w106) -> ("Width"=w111:u32, "Height"=w114:u32)
  n251 = control-ref of="Quit"() -> (w98:refnum<vi>)
  n252 = To Word Integer(number=w111) -> (16bit integer=w113:i16)
  n253 = To Word Integer(number=w114) -> ()  [unwired: 1 out]
  n254 = property class="Bool (strict)"(reference=w98) -> ("Height"=w116:u32, "Top"=w117:i32)  [unwired: 1 in, 2 out]
  n255 = Unbundle By Name(w108) -> ("Left"=w110:i16, "Top"=w121:i16)
  n256 = To Word Integer(number=w116) -> (16bit integer=w119:i16)
  n257 = To Word Integer(number=w117) -> (16bit integer=w120:i16)
  n258 = Add(x=w110, y=w113) -> (x+y=w112:i16)
  n259 = Compound Arithmetic op=ADD(w121, w119, w120, i16 12 ("y")) -> (w115:i16)
  n260 = Bundle By Name(cluster=w108, "Right"=w112, "Bottom"=w115) -> (w109:T21)
  n261 = property class="VI"(reference=w107, "Front Panel.PanelBounds"=w109) -> ()  [unwired: 1 in, 2 out]
